vi "tm3samp_sequence_polling.vi"() -> ()   [LabVIEW 2011]
panel:
  out "Counter":i32
  out "Image":u16[][](graph)
  out "Frames Per Second":dbl
  in  "Quit":bool
  out "Error Out":errorcluster
  # "This is an example of how to check\nfor a new frame instead of waiting\nfor a new frame.  The counter will\nupdate while waiting for a new\nframe to arrive."
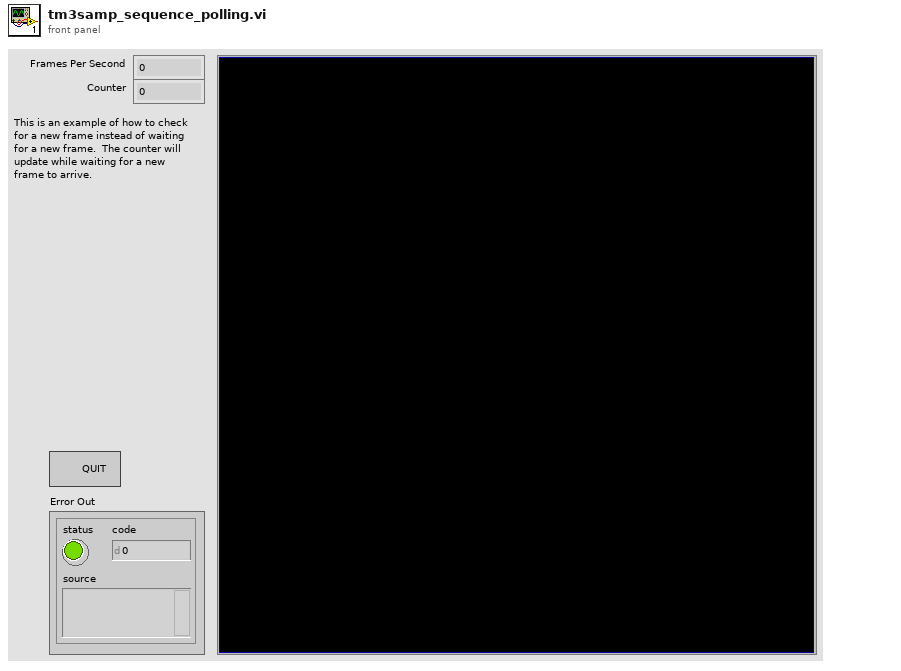
[diagram p1: front panel]
types:
  T1 = cluster{"width":u32, "height":u32, "datatype":u32}
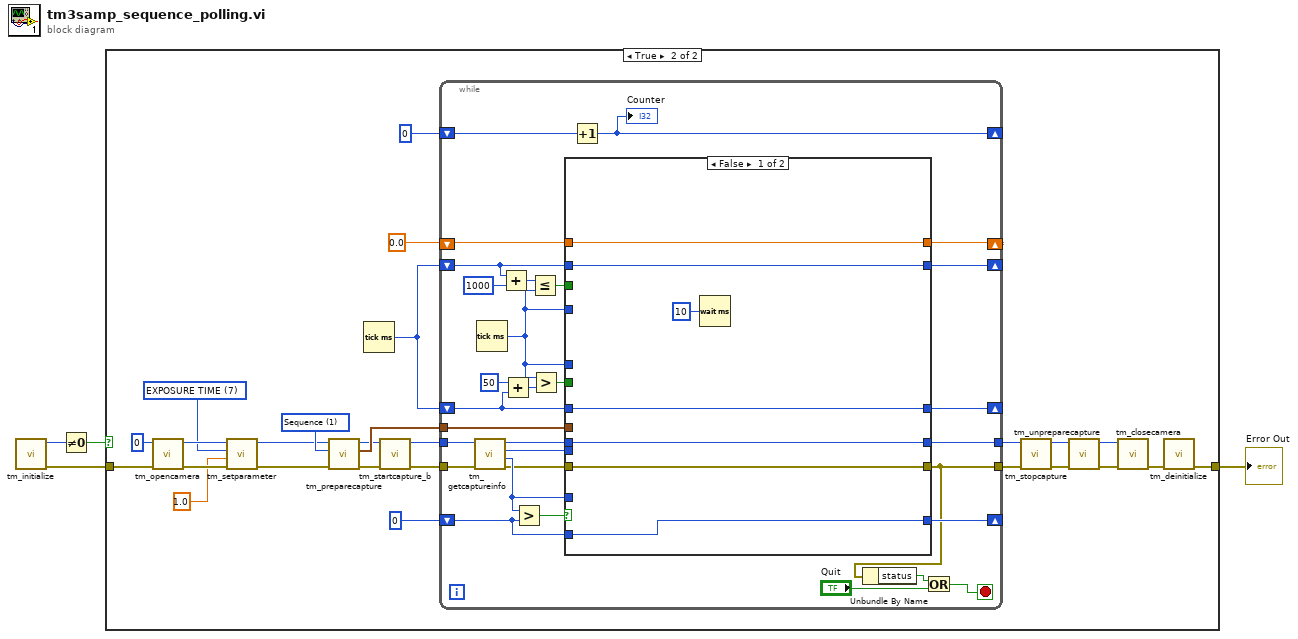
[diagram p0: block diagram]
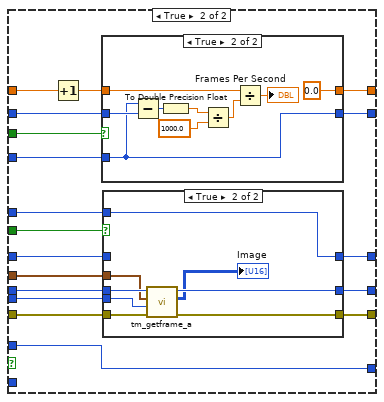
[diagram p3: hidden frame]
diagram:
  n1 = call <userlib>:"tm_initialize.vi"() -> ("error out"=w1:errorcluster, "Number Of Cameras"=w2:u32)  [unwired: 10 in]
  n2 = Not Equal To 0?(x=w2) -> (x != 0?=w4:bool)
  n3 = case shown="True" w4 {
    tunnel: w1 -> [w5 w31]
    tunnel: [w5 w27] -> w3
    frame False {
    }
    frame True {
      w8 = 7 items=["BINNING"=1, "BITS PER CHANNEL"=2, "ACTIVE VIEW INDEX"=3, "CCD MODE"=4, "SENSOR MODE"=5, "READOUT MODE"=6, "EXPOSURE TIME"=7, "CONTRAST GAIN"=8, "CONTRAST OFFSET"=9, "LIGHT MODE"=10, "SENSITIVITY"=11, "WHITE BALANCE"=12, "PHOTON IMAGING MODE"=13, "HIGH DYNAMIC RANGE MODE"=14, "TRIGGER SOURCE"=15, "TRIGGER ACTIVE"=16, "TRIGGER MODE"=17, "TRIGGER POLARITY"=18, "TRIGGER GLOBAL EXPOSURE"=19, "FIRST TRIGGER BEHAVIOR"=20, "TRIGGER TIMES"=21, "OUTPUT TRIGGER POLARITY"=22, "OUTPUT TRIGGER DELAY"=23, "OUTPUT TRIGGER PERIOD"=24, "TEMPERATURE"=25, "TEMPERATURE TARGET"=26, "SENSOR COOLER FAN"=27, "MECHANICAL SHUTTER"=28, "BACK FOCUS POSITION"=29, "FRAMEBUNDLE MODE"=30, "FRAMEBUNDLE NUMBER"=31, "LINEBUNDLE HEIGHT"=32, "TRIGGER CONNECTOR"=33, "IMAGE PIXEL TYPE"=34, "OUTPUT TRIGGER KIND"=35, "READOUT DIRECTION"=36] ("Parameter")
      w29 = 1 items=["Snap", "Sequence"] ("Capture mode")
      n4 = call <userlib>:"tm_opencamera.vi"("error in (no error)"=w31, "Camera Index"=u32 0) -> ("error out"=w9:errorcluster, "Handle out"=w12:u32)  [unwired: 8 in]
      n5 = call <userlib>:"tm_setparameter.vi"("error in (no error)"=w9, "Value in"=1.0, "Parameter"=w8, "Handle in"=w12) -> ("error out"=w10:errorcluster, "Handle out"=w11:u32)  [unwired: 6 in]
      n6 = call <userlib>:"tm_preparecapture.vi"("error in (no error)"=w10, "Capture mode"=w29, "Handle in"=w11) -> ("error out"=w19:errorcluster, "Buffer"=w24:T1, "Handle out"=w18:u32)  [unwired: 5 in, 1 out]
      n7 = Tick Count (ms)() -> (millisecond timer value=w14:u32)
      n8 = call <userlib>:"tm_startcapture_b.vi"("error in (no error)"=w19, "Handle in"=w18) -> ("error out"=w16:errorcluster, "Handle out"=w17:u32)  [unwired: 8 in]
      n9 = while {
        tunnel: [w50] -> w22
        tunnel: [w49] -> w23
        tunnel: w24 -> [w48]
        tunnel: w17 -> [w57]
        tunnel: w16 -> [w56]
        shift-right: [w55] -> _
        shift-left: 0 -> [w54]
        shift-right: [w46] -> _
        shift-left: w14 -> [w34]
        shift-right: [w47] -> _
        shift-left: w14 -> [w35]
        shift-right: [w44] -> _
        shift-left: 0.0 -> [w45]
        shift-right: [w32] -> _
        shift-left: 0 -> [w33]
        stop <- w43 stop-if-true
        n10 = call <userlib>:"tm_getcaptureinfo.vi"("error in (no error)"=w56, "Handle in"=w57) -> ("error out"=w52:errorcluster, "Frame Count"=w58:i32, "Frame Index"=w51:i32, "Handle out"=w53:u32)  [unwired: 6 in]
        n11 = Tick Count (ms)() -> (millisecond timer value=w38:u32)
        n12 = Add(x=w34, y=u32 1000) -> (x+y=w39:u32)
        n13 = Add(x=u32 50, y=w35) -> (x+y=w42:u32)
        n14 = Greater?(x=w58, y=w54) -> (0:w59:bool)
        n15 = Less Or Equal?(x=w39, y=w38) -> (x <= y?=w36:bool)
        n16 = Greater?(x=w38, y=w42) -> (0:w37:bool)
        n17 = case shown="False" w59 {
          tunnel: w54 -> [w68 _]
          tunnel: [w68 w71] -> w55
          tunnel: w58 -> [_ w71]
          tunnel: w53 -> [w66 w86]
          tunnel: w52 -> [w67 w84]
          tunnel: w51 -> [_ w85]
          tunnel: [w67 w79] -> w49
          tunnel: [w66 w80] -> w50
          tunnel: w48 -> [_ w83]
          tunnel: w34 -> [w64 w82]
          tunnel: w35 -> [w65 w81]
          tunnel: [w65 w78] -> w47
          tunnel: [w64 w77] -> w46
          tunnel: w45 -> [w63 w69]
          tunnel: [w63 w76] -> w44
          tunnel: w38 -> [_ w75]
          tunnel: w38 -> [_ w74]
          tunnel: w37 -> [_ w73]
          tunnel: w36 -> [_ w72]
          frame False {
            n18 = Wait (ms)(milliseconds to wait=u32 10) -> ()  [unwired: 1 out]
          }
          frame True {
            n19 = Increment(x=w69) -> (x+1=w70:dbl)
            n20 = case shown="True" w72 {
              tunnel: w82 -> [w99 w102]
              tunnel: [w99 w100] -> w77
              tunnel: w70 -> [w98 w106]
              tunnel: w75 -> [_ w100]
              tunnel: [w98 0.0] -> w76
              frame False {
              }
              frame True {
                n21 = Subtract(x=w100, y=w102) -> (x-y=w101:u32)
                n22 = To Double Precision Float(number=w101) -> (double precision float=w108:dbl)
                n23 = Divide(x=w108, y=1000.0) -> (x/y=w105:dbl)
                n24 = Divide(x=w106, y=w105) -> (x/y=→"Frames Per Second":dbl)
              }
            }
            n25 = case shown="True" w73 {
              tunnel: w86 -> [w89 w97]
              tunnel: w84 -> [w88 w96]
              tunnel: w85 -> [_ w95]
              tunnel: w81 -> [w87 _]
              tunnel: w74 -> [_ w94]
              tunnel: [w89 w91] -> w80
              tunnel: [w88 w92] -> w79
              tunnel: [w87 w94] -> w78
              tunnel: w83 -> [_ w93]
              frame False {
              }
              frame True {
                n26 = call <userlib>:"tm_getframe_a.vi"("error in (no error)"=w96, "Frame Index"=w95, "Buffer"=w93, "Handle in"=w97) -> ("error out"=w92:errorcluster, "Data 16"=→"Image":u16[][], "Handle out"=w91:u32)  [unwired: 3 in, 2 out]
              }
            }
          }
        }
        n27 = Increment(x=w33) -> (x+1=w32:i32)
        "Counter" <- w32
        n28 = Unbundle By Name(w49) -> ("status"=w61:bool)
        n29 = Or(x=w61, y="Quit") -> (x .or. y?=w43:bool)
      }
      n30 = call <userlib>:"tm_stopcapture.vi"("error in (no error)"=w23, "Handle in"=w22) -> ("error out"=w20:errorcluster, "Handle out"=w21:u32)  [unwired: 8 in]
      n31 = call <userlib>:"tm_unpreparecapture.vi"("error in (no error)"=w20, "Handle in"=w21) -> ("error out"=w26:errorcluster, "Handle out"=w25:u32)  [unwired: 8 in]
      n32 = call <userlib>:"tm_closecamera.vi"("error in (no error)"=w26, "Handle in"=w25) -> ("error out"=w28:errorcluster)  [unwired: 9 in]
      n33 = call <userlib>:"tm_deinitialize.vi"("error in (no error)"=w28) -> ("error out"=w27:errorcluster)  [unwired: 10 in]
    }
  }
  "Error Out" <- w3
